vi "Test Init from Node-ID.vi"(11 "Test Case In":refnum<class "Test CANopen Message.lvclass">) -> (0 "error out":errorcluster, 3 "Test Case Out":refnum<class "Test CANopen Message.lvclass">)   [LabVIEW 2024, in "Test CANopen Message.lvclass"]
uses:
  Test CANopen Message.lvclass
  C:/Program Files/National Instruments/LabVIEW 2026/vi.lib/Astemes/LUnit/Test Case.lvclass
  CANopen Message/CANopen Message.lvclass/CANopen Message.ctl
  <vilib>/Astemes/LUnit/Test Case.lvclass/Test Case.ctl
  CANopen Message/CANopen Message.lvclass
  Test CANopen Message.lvclass/Test CANopen Message.ctl
  C:/Program Files/National Instruments/LabVIEW 2026/vi.lib/Astemes/LUnit/LUnit Runnable.lvclass
  D:/git/CANopen-LabVIEW/tests/Test CANopen Message/Test CANopen Message.lvclass
  source/Typedefs/Function Code.ctl
  source/CANopen.lvlib
  <vilib>/Astemes/LUnit/Test Case.lvclass
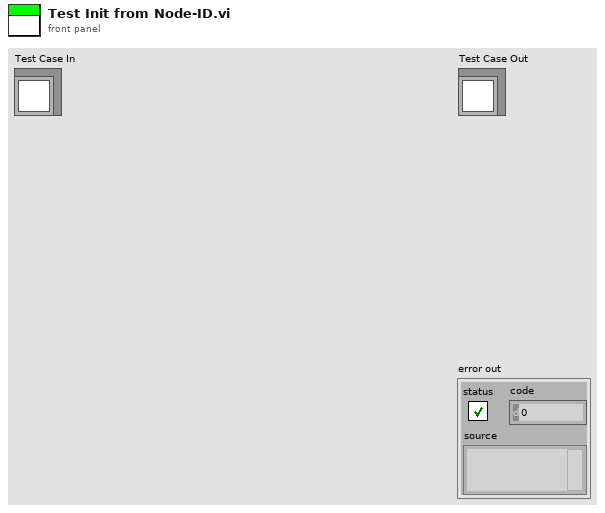
[diagram p1: front panel]
types:
  T1 = typedef "CANopen.lvlib/Function Code.ctl" = u8
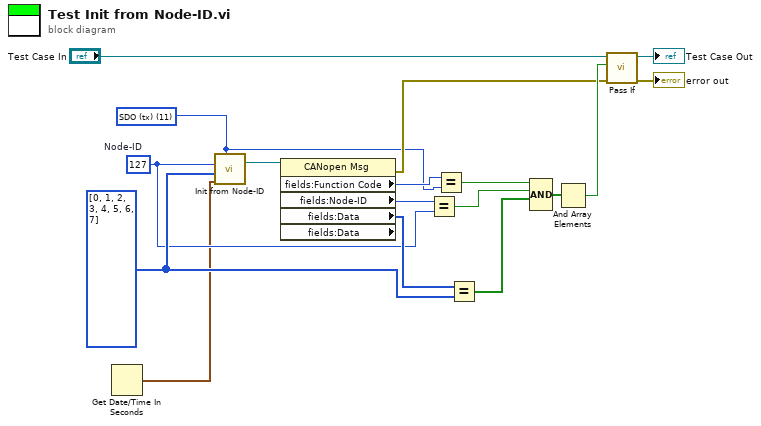
[diagram p0: block diagram]
diagram:
  w2 = T1 11 items=["NMT"=0, "EMCY/SYNC"=1, "TIME"=2, "PDO1 (tx)"=3, "PDO1 (rx)"=4, "PDO2 (tx)"=5, "PDO2 (rx)"=6, "PDO3 (tx)"=7, "PDO3 (rx)"=8, "PDO4 (tx)"=9, "PDO4 (rx)"=10, "SDO (tx)"=11, "SDO (rx)"=12, "NMT error control"=14] ("Function Code")
  w10 = u8[] [0, 1, 2, 3, 4, 5, 6, 7] ("Data")
  w9 = u8 127  # Node-ID
  n1 = Get Date/Time In Seconds() -> (seconds since 1Jan1904=w1:timestamp)
  n2 = call "Init from Node-ID.vi"("Function Code"=w2, "Timestamp"=w1, "Data"=w10, "Node-ID"=w9) -> ("CANopen Message"=w14:refnum<class "CANopen Message.lvclass">)  [unwired: 7 in]
  n3 = property class="CANopen Msg" props=["fields:Function Code", "fields:Node-ID", "fields:Data", "fields:Data"](reference=w14) -> (error out=w3:errorcluster, "fields:Function Code"=w12:T1, "fields:Node-ID"=w13:u8, "fields:Data"=w11:u8[])  [unwired: 1 in, 2 out]
  n4 = Equal?(x=w13, y=w9) -> (x = y?=w7:bool)
  n5 = Equal?(x=w12, y=w2) -> (x = y?=w8:bool)
  n6 = Equal?(x=w11, y=w10) -> (x = y?=w6:bool[])
  n7 = Compound Arithmetic op=AND(w8, w7, w6) -> (w5:bool[])  [unwired: 1 in]
  n8 = And Array Elements(Boolean array=w5) -> (logical AND=w4:bool)
  n9 = call <vilib>:"Pass If.vi"("error in (no error)"=w3, "Pass?"=w4, "LUnit Test Case In"="Test Case In") -> ("error out"=→"error out":errorcluster, "LUnit Test Case Out"=→"Test Case Out":refnum<class "Test CANopen Message.lvclass">)  [unwired: 7 in]
